vi "ReadSudoku.vi"(11 "Jpeg path":path) -> (0 "error out":errorcluster, 2 "image data":T1, 3 "Picture":picture)   [LabVIEW 2020]
uses:
  <vilib>/picture/picture.llb/imagedata.ctl
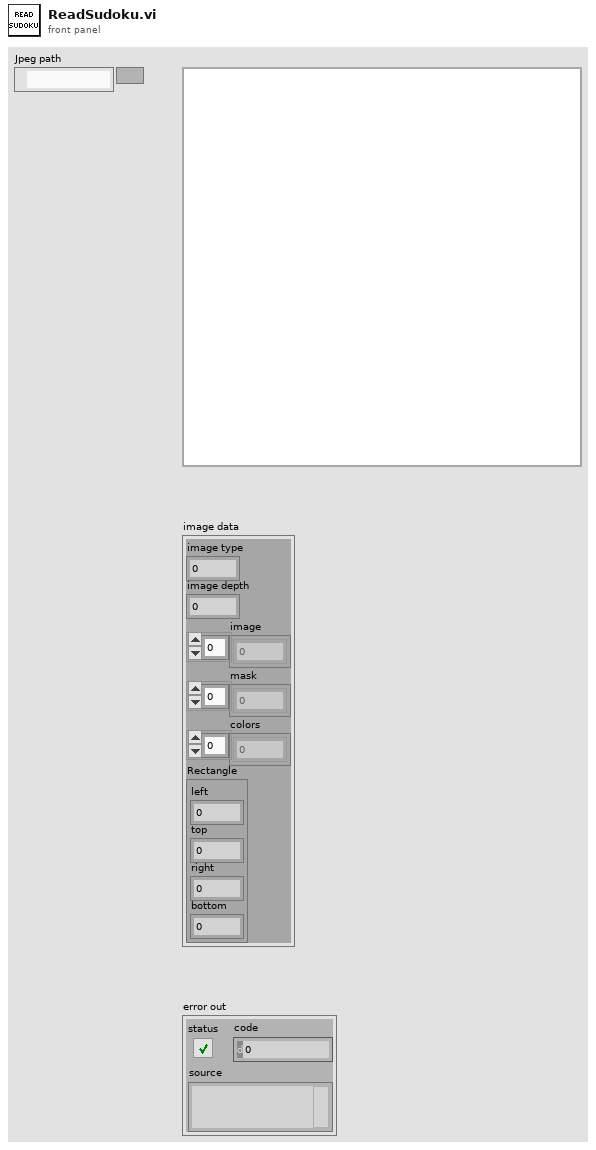
[diagram p1: front panel]
types:
  T1 = typedef "imagedata.ctl" = cluster{"image type":i32, "image depth":i32, "image":u8[], "mask":u8[], "colors":u32[], "Rectangle":cluster{"left":i16, "top":i16, "right":i16, "bottom":i16}}
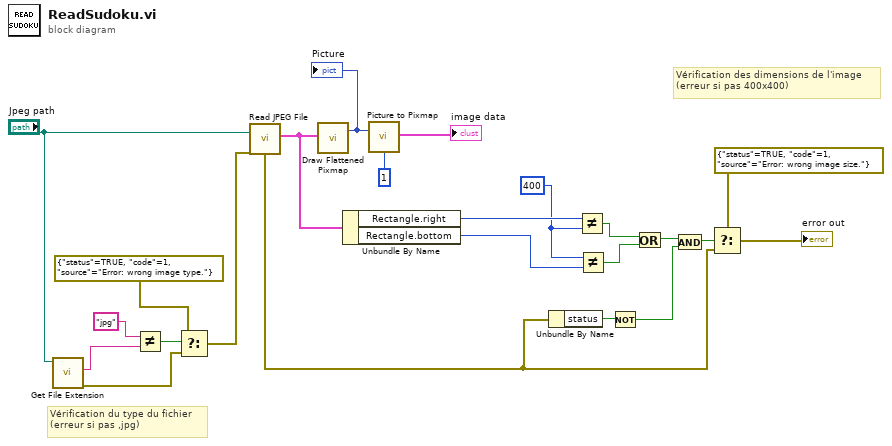
[diagram p0: block diagram]
diagram:
  w17 = 400
  # "Vérification des dimensions de l'image\n(erreur si pas 400x400)"
  # "Vérification du type du fichier\n(erreur si pas ,jpg)"
  n1 = call <vilib>:"Get File Extension.vi"("file"="Jpeg path") -> ("error out"=w8:errorcluster, "lowercase file extension"=w11:string)  [unwired: 6 in, 3 out]
  n2 = Not Equal?(x="jpg", y=w11) -> (x != y?=w9:bool)
  n3 = Select(t=errorcluster {"status"=TRUE, "code"=1, "source"="Error: wrong image type."}, s=w9, f=w8) -> (s? t:f=w6:errorcluster)
  n4 = call <vilib>:"Read JPEG File.vi"("error in (no error)"=w6, "path to JPEG file"="Jpeg path") -> ("error out"=w5:errorcluster, "image data"=w20:T1)  [unwired: 7 in, 1 out]
  n5 = call <vilib>:"Draw Flattened Pixmap.vi"("image data"=w20) -> ("new picture"=w23:picture)  [unwired: 8 in]
  "Picture" <- w23
  n6 = Unbundle By Name(w20) -> ("Rectangle.right"=w19:i16, "Rectangle.bottom"=w18:i16)
  n7 = call <vilib>:"Picture to Pixmap.vi"("depth"=1, "picture"=w23) -> ("image data"=→"image data":T1)  [unwired: 8 in, 1 out]
  n8 = Unbundle By Name(w5) -> ("status"=w4:bool)
  n9 = Not Equal?(x=w19, y=w17) -> (x != y?=w16:bool)
  n10 = Not Equal?(x=w17, y=w18) -> (x != y?=w15:bool)
  n11 = Not(x=w4) -> (.not. x?=w1:bool)
  n12 = Or(x=w16, y=w15) -> (x .or. y?=w2:bool)
  n13 = And(x=w2, y=w1) -> (x .and. y?=w3:bool)
  n14 = Select(t=errorcluster {"status"=TRUE, "code"=1, "source"="Error: wrong image size."}, s=w3, f=w5) -> (s? t:f=→"error out":errorcluster)
